vi "Database-AddComponent.vi"(7 "Idx":i32, 8 "error in":errorcluster, 9 "Product Component":T1) -> (0 "error out":errorcluster)   [LabVIEW 2016]
doc: "Go to DB->WriteStationValues action\nReturn boolean flag to show if data was saved to DB successfully\n\nWabco 2017 All right reserved\nAuthor: maciej.szupienko@wabco-auto.com"
uses:
  ProdaNG/Controls/ProdaNG.ProductComponent.ctl
  Database.Action.ctl
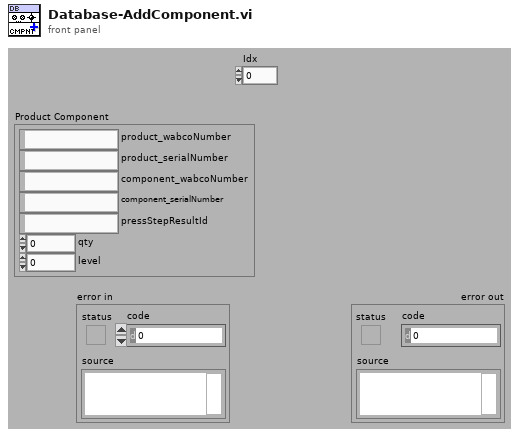
[diagram p1: front panel]
types:
  T1 = typedef "ProdaNG.ProductComponent.ctl" = cluster{"product_wabcoNumber":string, "product_serialNumber":string, "component_wabcoNumber":string, "component_serialNumber":string, "pressStepResultId":string, "qty":i32, "level":i32}
  T2 = typedef "Database.Action.ctl" = enum32{"idle", "constructor", "destructor", "--- DB ---", "Setup", "Disconnect", "Connect", "GetAllStatuses"}
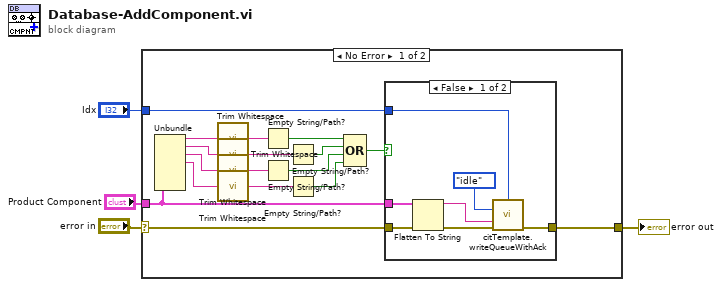
[diagram p0: block diagram]
diagram:
  n1 = case shown="No Error" "error in" {
    selector: "error in" -> [w20 w30]
    tunnel: [w19 w30] -> w3
    tunnel: "Idx" -> [w21 _]
    tunnel: "Product Component" -> [w18 _]
    frame No Error {
      n2 = Unbundle(w18) -> ("product_wabcoNumber"=w13:string, "product_serialNumber"=w12:string, "component_wabcoNumber"=w11:string, "component_serialNumber"=w10:string)  [unwired: 3 out]
      n3 = call <vilib>:"Trim Whitespace.vi"("string"=w13) -> ("trimmed string"=w8:string)  [unwired: 1 in]
      n4 = call <vilib>:"Trim Whitespace.vi"("string"=w12) -> ("trimmed string"=w7:string)  [unwired: 1 in]
      n5 = call <vilib>:"Trim Whitespace.vi"("string"=w11) -> ("trimmed string"=w6:string)  [unwired: 1 in]
      n6 = call <vilib>:"Trim Whitespace.vi"("string"=w10) -> ("trimmed string"=w5:string)  [unwired: 1 in]
      n7 = Empty String/Path?(string/path=w8) -> (empty?=w17:bool)
      n8 = Empty String/Path?(string/path=w6) -> (empty?=w15:bool)
      n9 = Empty String/Path?(string/path=w7) -> (empty?=w16:bool)
      n10 = Empty String/Path?(string/path=w5) -> (empty?=w14:bool)
      n11 = Compound Arithmetic op=OR(w17, w16, w15, w14) -> (w9:bool)
      n12 = case shown="False" w9 {
        tunnel: w21 -> [w28 _]
        tunnel: w20 -> [w24 w29]
        tunnel: [w23 w29] -> w19
        tunnel: w18 -> [w22 _]
        frame False {
          n13 = Flatten To String(anything=w22, error in (no error)=w24) -> (data string=w25:string, error out=w27:errorcluster)  [unwired: 2 in, 1 out]
          n14 = call "citTemplate.writeQueueWithAck.vi"("instance (0)"=w28, "event in"=Database.Action."idle" ("Action"), "(flatten) data in"=w25, "error in (no error)"=w27) -> ("error out"=w23:errorcluster)  [unwired: 9 in, 2 out]
        }
        frame True {
        }
      }
    }
    frame Error {
    }
  }
  "error out" <- w3
